vi "Main.vi"(8 "error in":errorcluster, 9 ">>ErrorQ":refnum<queue>, 11 ">>EventHandlers":refnum<user-event>) -> (0 "error out":errorcluster)   [LabVIEW 2020, in "DisplayConsole.lvlib"]
doc: "This is a template for creating new VIs for the owning library"
uses:
  DisplayConsole.lvlib
  Error Handler/Controls/Error QMsg.ctl
  Support/Controls/Project Modules.ctl
  Support/Controls/Project Event Msg.ctl
  Support/Controls/Project Events.ctl
  Controls/Operational Loop Data.ctl
  Controls/Module QMsg.ctl
  Support/Support.lvlib
  Controls/Module Event Msg.ctl
  Error Handler/ErrorHandler.lvlib
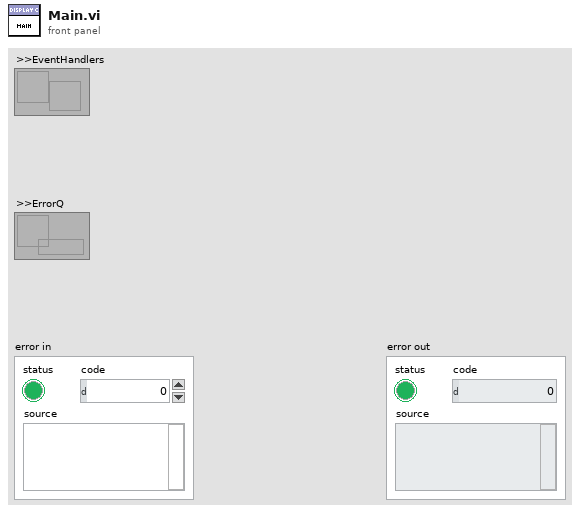
[diagram p1: front panel]
types:
  T1 = typedef "DisplayConsole.lvlib/Module QMsg.ctl" = cluster{"Command":string, "Data":variant}
  T2 = typedef "DisplayConsole.lvlib/Operational Loop Data.ctl" = cluster{"Dummy":dbl}
  T3 = typedef "DisplayConsole.lvlib/Module Messaging Structures.ctl" = cluster{">>EventHandlers":refnum<user-event>, ">>ErrorQ":refnum<queue>}
  T4 = typedef "DisplayConsole.lvlib/Module Event Msg.ctl" = cluster{"Command":string, "Data":variant}
  T5 = typedef "Support.lvlib/Project Events.ctl" = enum16{"Stop", "Initialize", "Elevator Call"}
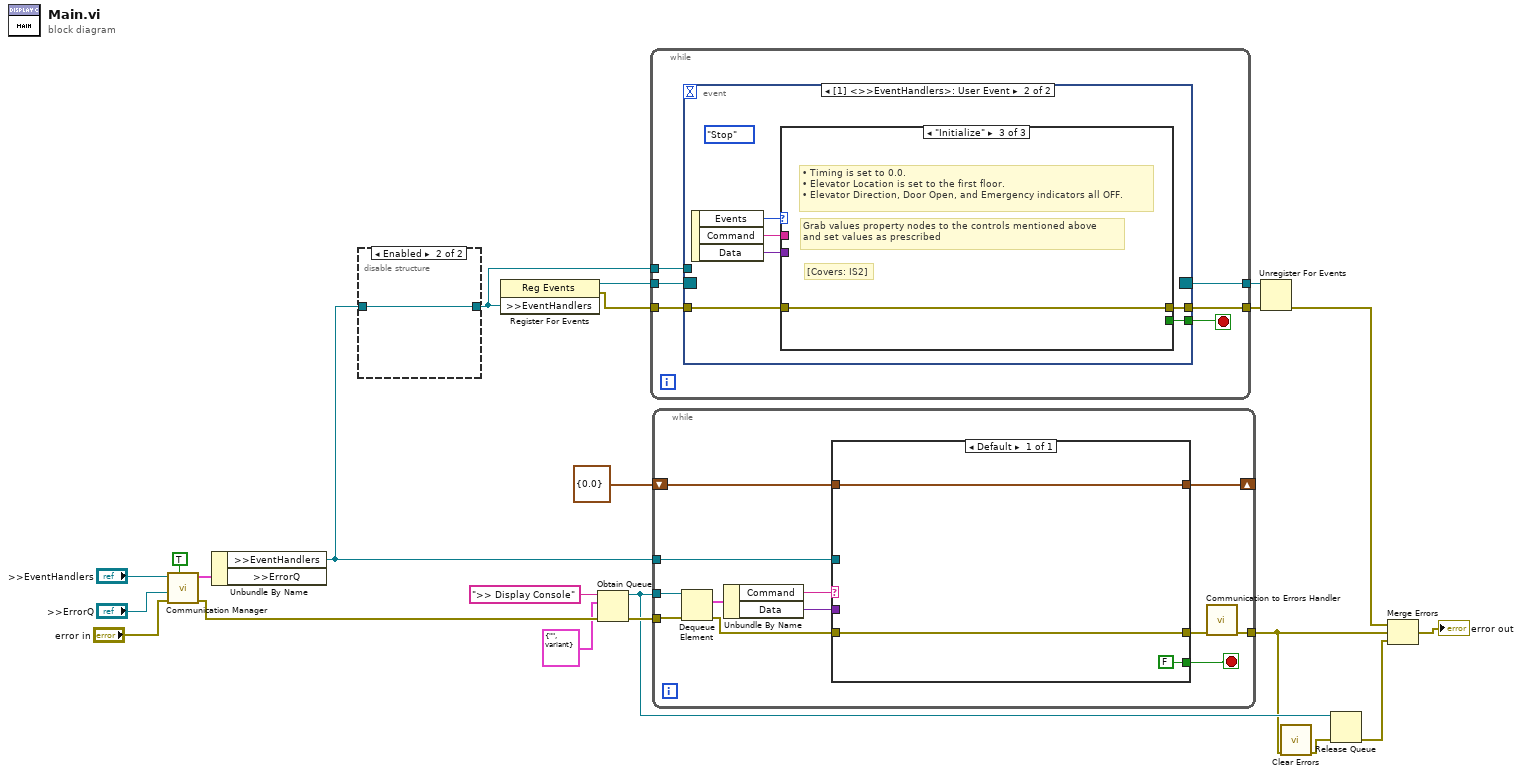
[diagram p0: block diagram]
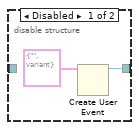
[diagram p2: hidden frame]
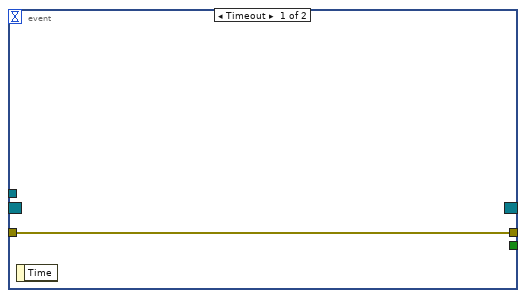
[diagram p3: hidden frame]
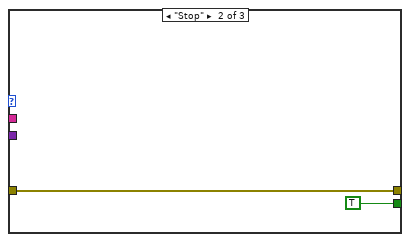
[diagram p5: hidden frame]
diagram:
  n1 = call "Communication Manager.vi"("Load?"=TRUE, "error in"="error in", ">>ErrorQ"=">>ErrorQ", ">>EventHandlers"=">>EventHandlers") -> ("error out"=w8:errorcluster, "Messaging Structures"=w18:T3)  [unwired: 6 in]
  n2 = Unbundle By Name(w18) -> (">>EventHandlers"=w11:refnum<user-event>)  [unwired: 1 out]
  n3 = disable-structure shown="Enabled" {
    disable-tunnel: w11 -> [_ w25]
    disable-tunnel: [w23 w25] -> w10
    frame Disabled {
      n4 = Create User Event(user event datatype=T4 {"Command"="", "Data"=variant} ("QMessage")) -> (user event=w23:refnum<user-event>)  [unwired: 1 in, 1 out]
    }
    frame Enabled {
    }
  }
  n5 = register-events(w10) -> (reference out=w17:refnum<event-registration>, error out=w15:errorcluster)  [unwired: 2 in]
  n6 = Obtain Queue(name (unnamed)=">> Display Console", element data type=T1 {"Command"="", "Data"=variant} ("QMessage"), error in (no error)=w8) -> (queue out=w3:refnum<queue>, error out=w9:errorcluster)  [unwired: 2 in, 1 out]
  n7 = while {
    tunnel: w10 -> [w31]
    tunnel: w17 -> [w30]
    tunnel: [w29] -> w16
    tunnel: w15 -> [w28]
    tunnel: [w27] -> w14
    stop <- w26 stop-if-true
    n8 = event shown="[1] <>>EventHandlers>: User Event" {
      selector: w30 -> [_ _]
      dyn-events: [_ _] -> w29
      timeout: _ -> [_ _]
      tunnel: w31 -> [_ _]
      tunnel: w28 -> [w32 w38]
      tunnel: [w32 w37] -> w27
      tunnel: [_ w35] -> w26
      event Timeout {
        n9 = event-data() -> ()  [unwired: 1 in, 1 out]
      }
      event User Event {
        (unwired) Project_Events."Stop" ("Events")
        n10 = event-data() -> ("Events"=w36:T5, "Command"=w34:string, "Data"=w33:variant)  [unwired: 1 in]
        n11 = case shown="\"Initialize\"" w36 {
          tunnel: w38 -> [w39 w41 w42]
          tunnel: [w39 w41 w42] -> w37
          tunnel: [_ TRUE _] -> w35
          tunnel: w34 -> [_ _ _]
          tunnel: w33 -> [_ _ _]
          frame Default {
          }
          frame "Stop" {
          }
          frame "Initialize" {
            # "[Covers: IS2]"
            # "Grab values property nodes to the controls mentioned above\nand set values as prescribed"
            # "• Timing is set to 0.0.\n• Elevator Location is set to the first floor.\n• Elevator Direction, Door Open, and Emergency indicators all OFF."
          }
        }
      }
    }
  }
  n12 = while {
    tunnel: w3 -> [w54]
    tunnel: w11 -> [w47]
    tunnel: w9 -> [w53]
    tunnel: [w45] -> w2
    shift-right: [w43] -> _
    shift-left: T2 {"Dummy"=0.0} ("Operation Loop Data") -> [w44]
    stop <- w49 stop-if-true
    n13 = Dequeue Element(queue=w54, error in (no error)=w53) -> (element=w52:T1, error out=w48:errorcluster)  [unwired: 1 in, 2 out]
    n14 = Unbundle By Name(w52) -> ("Command"=w51:string, "Data"=w50:variant)
    n15 = case shown="Default" w51 {
      tunnel: w50 -> [_]
      tunnel: [FALSE] -> w49
      tunnel: w48 -> [w57]
      tunnel: [w57] -> w46
      tunnel: w47 -> [_]
      tunnel: w44 -> [w56]
      tunnel: [w56] -> w43
      frame Default {
      }
    }
    n16 = call "Communication to Errors Handler.vi"("error in"=w46) -> ("error out"=w45:errorcluster)  [unwired: 10 in]
  }
  n17 = Unregister For Events(event registration refnum=w16, error in=w14) -> (error out=w13:errorcluster)
  n18 = call <vilib>:"Clear Errors.vi"("error in (no error)"=w2) -> ("error out"=w4:errorcluster)  [unwired: 5 in, 1 out]
  n19 = Release Queue(queue=w3, error in (no error)=w4) -> (error out=w1:errorcluster)  [unwired: 1 in, 2 out]
  n20 = Merge Errors(w13, w2, w1) -> (→"error out":errorcluster)
